vi "fuzz.vi"() -> ()   [LabVIEW 2025]
panel:
  in  "Boolean 4":bool
  out "output array 6":dbl[][](array[numeric])
  out "output array 5":dbl[][](array[numeric])
  out "output array 4":dbl[][](array[numeric])
  out "output array 3":dbl[][](array[numeric])
  out "output array 2":dbl[][](array[numeric])
  out "output array":dbl[][](array[numeric])
  out "1-D Array of Real":dbl[](array[numeric])
  in  "stop 2":bool
  in  "Boolean 3":bool
  in  "Boolean 2":bool
  in  "Boolean":bool
  out "String 6":string
  out "String 5":string
  out "String 4":string
  out "String 3":string
  out "String 2":string
  out "IM6":picture
  out "IM5":picture
  out "IM4":picture
  out "IM3":picture
  out "IM2":picture
  out "Numeric":i32
  out "Real":dbl
  out "String":string
  out "?":picture
  in  "Evaluate":path
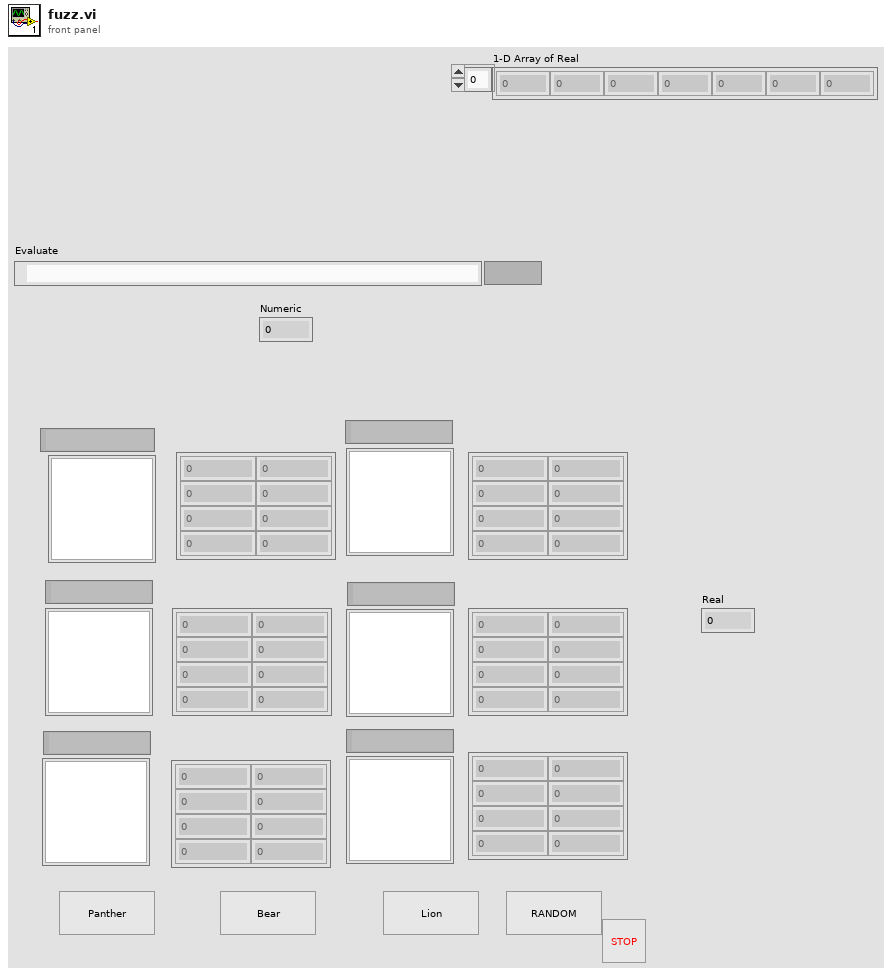
[diagram p1: front panel]
types:
  T1 = typedef "imagedata.ctl" = cluster{"image type":i32, "image depth":i32, "image":u8[], "mask":u8[], "colors":u32[], "Rectangle":cluster{"left":i16, "top":i16, "right":i16, "bottom":i16}}
  T2 = typedef "LVBoundsTypeDef.ctl" = cluster{"Width":u32, "Height":u32}
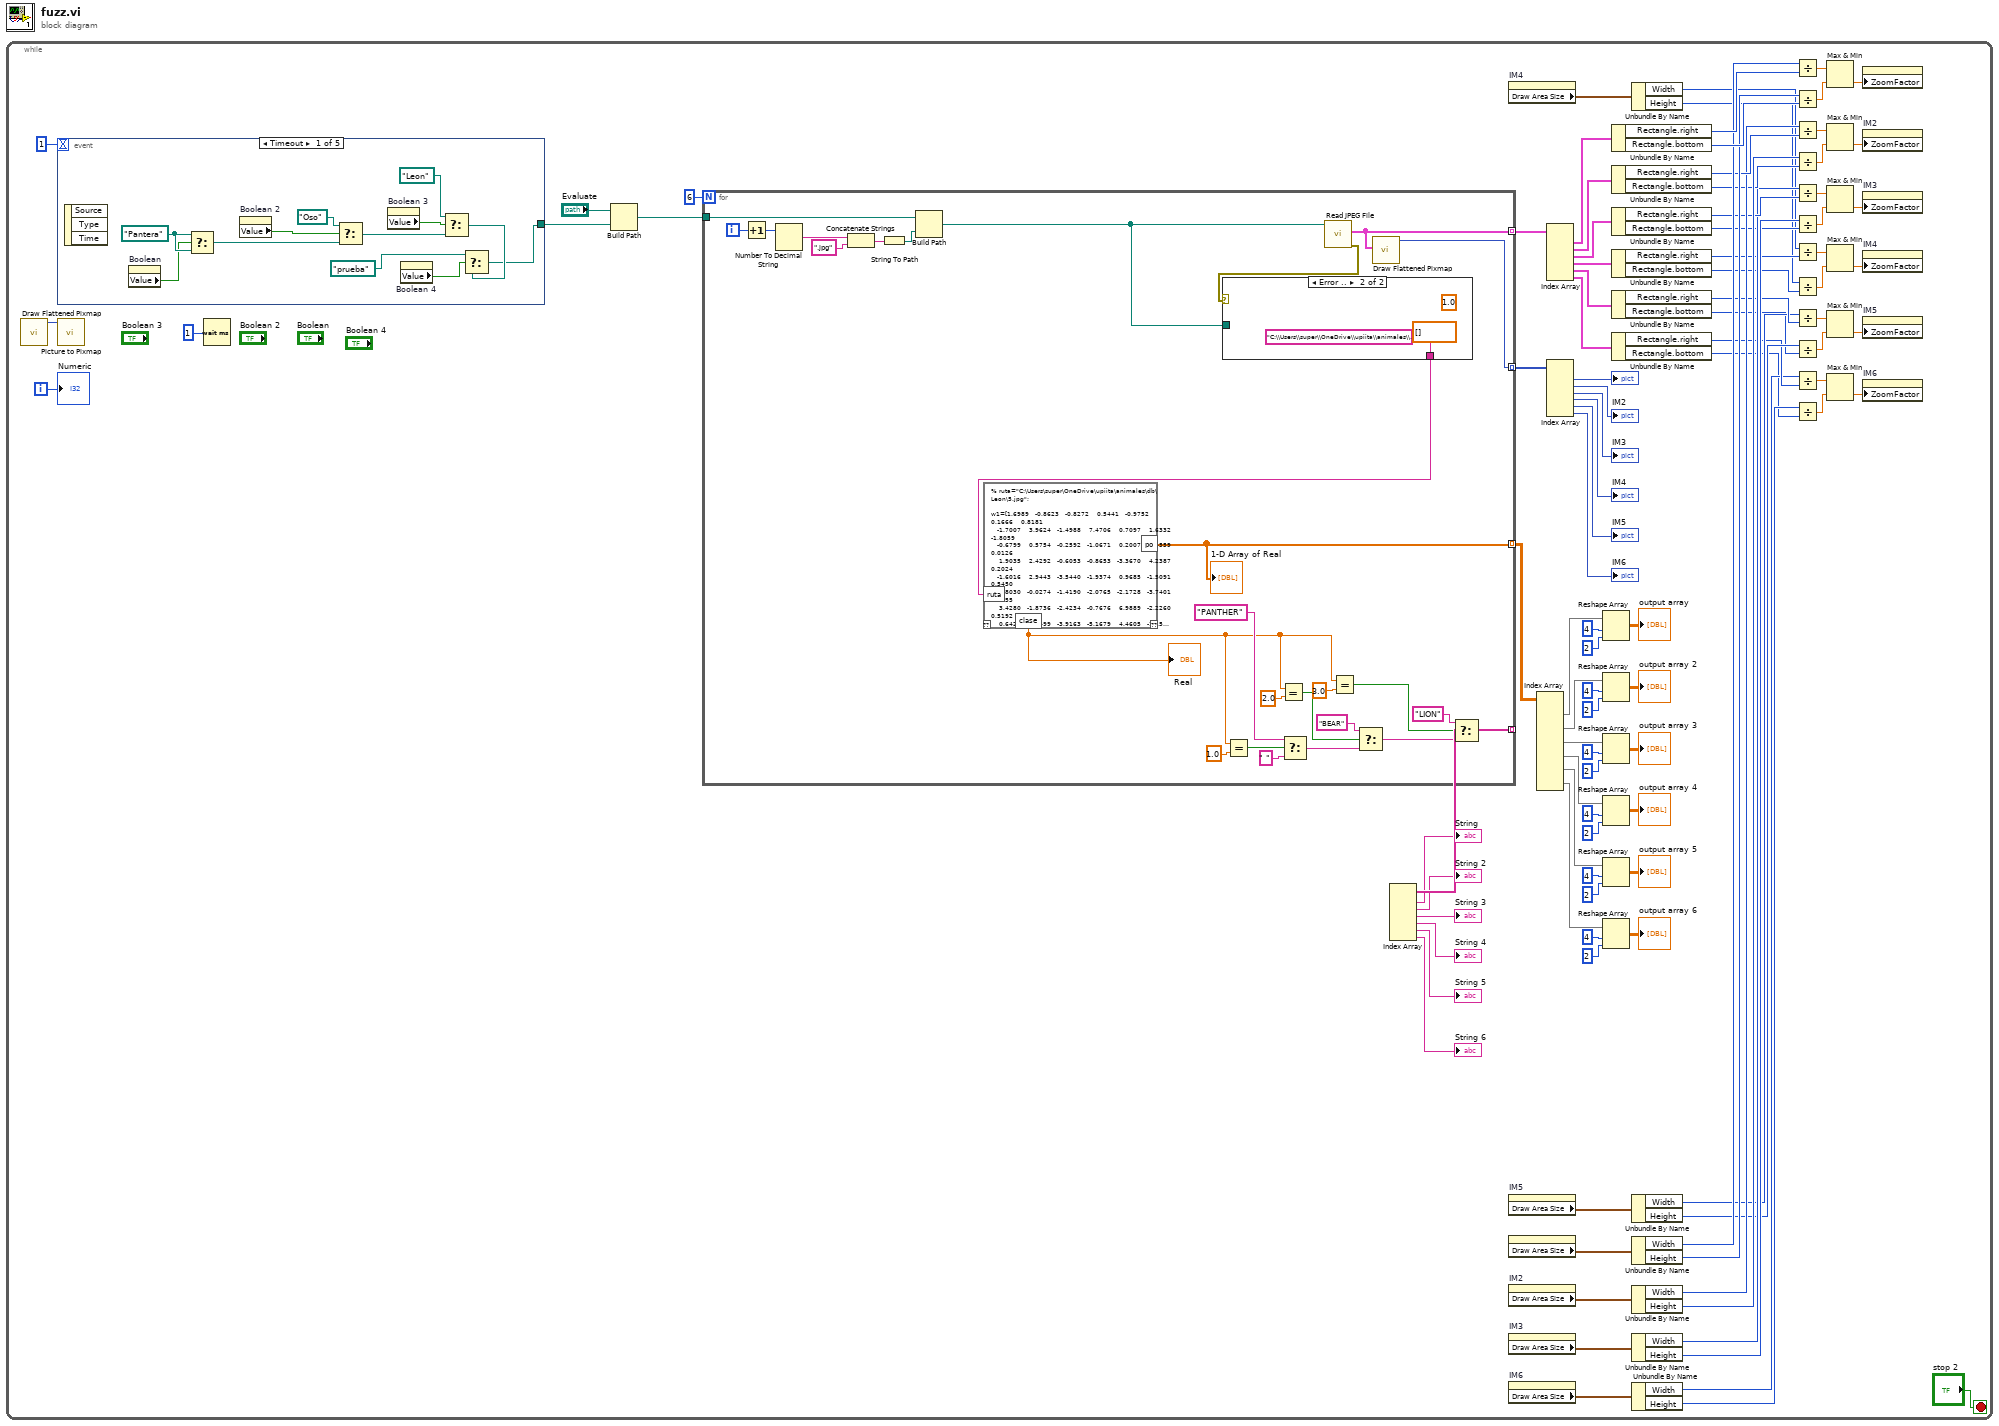
[diagram p0: block diagram]
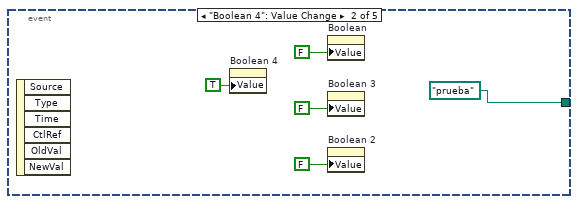
[diagram p2: hidden frame]
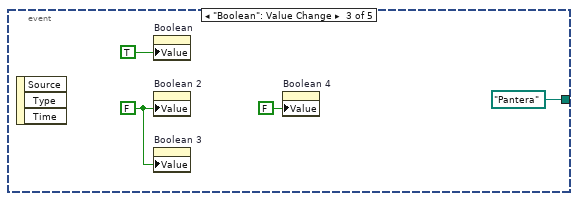
[diagram p3: hidden frame]
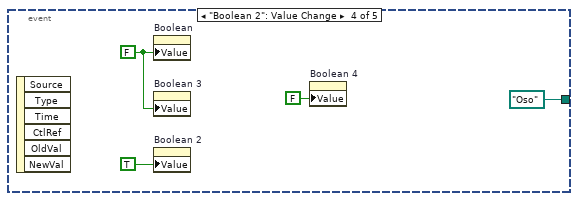
[diagram p4: hidden frame]
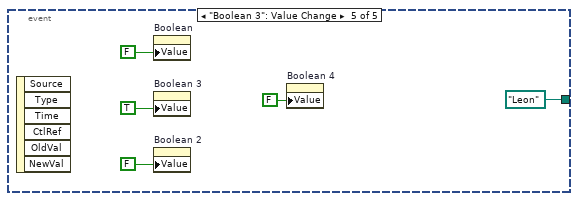
[diagram p5: hidden frame]
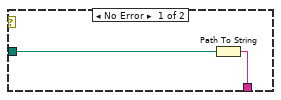
[diagram p6: hidden frame]
diagram:
  n1 = while {
    i -> [w103]
    stop <- "stop 2" stop-if-true
    n2 = call <vilib>:"Draw Flattened Pixmap.vi"() -> ("new picture"=w95:picture)  [unwired: 9 in]
    n3 = event shown="[0] Timeout" {
      selector: _ -> [_ _ _ _ _]
      dyn-events: _ -> [_ _ _ _ _]
      timeout: 1 -> [_ _ _ _ _]
      tunnel: [w104 path "prueba" ("Evaluate") path "Pantera" ("Evaluate") path "Oso" ("Evaluate") path "Leon" ("Evaluate")] -> w28
      event Timeout {
        w109 = path "Pantera" ("Evaluate")
        n4 = event-data() -> ()  [unwired: 1 in, 3 out]
        n5 = property on="Boolean" class="Bool (strict)"() -> ("Value"=w108:bool)  [unwired: 2 in, 2 out]
        n6 = Select(t=w109, s=w108, f=w109) -> (s? t:f=w113:path)
        n7 = property on="Boolean 2" class="Bool (strict)"() -> ("Value"=w112:bool)  [unwired: 2 in, 2 out]
        n8 = Select(t=path "Oso" ("Evaluate"), s=w112, f=w113) -> (s? t:f=w115:path)
        n9 = property on="Boolean 3" class="Bool (strict)"() -> ("Value"=w114:bool)  [unwired: 2 in, 2 out]
        n10 = property on="Boolean 4" class="Bool (strict)"() -> ("Value"=w107:bool)  [unwired: 2 in, 2 out]
        n11 = Select(t=path "Leon" ("Evaluate"), s=w114, f=w115) -> (s? t:f=w105:path)
        n12 = Select(t=path "prueba" ("Evaluate"), s=w107, f=w105) -> (s? t:f=w104:path)
      }
      event "Boolean 4": Value Change {
        n13 = event-data() -> ()  [unwired: 1 in, 6 out]
        n14 = property on="Boolean 4" class="Bool (strict)"("Value"=TRUE ("Boolean 4")) -> ()  [unwired: 2 in, 2 out]
        n15 = property on="Boolean" class="Bool (strict)"("Value"=FALSE) -> ()  [unwired: 2 in, 2 out]
        n16 = property on="Boolean 3" class="Bool (strict)"("Value"=FALSE) -> ()  [unwired: 2 in, 2 out]
        n17 = property on="Boolean 2" class="Bool (strict)"("Value"=FALSE) -> ()  [unwired: 2 in, 2 out]
      }
      event "Boolean": Value Change {
        w124 = FALSE
        n18 = event-data() -> ()  [unwired: 1 in, 3 out]
        n19 = property on="Boolean" class="Bool (strict)"("Value"=TRUE) -> ()  [unwired: 2 in, 2 out]
        n20 = property on="Boolean 2" class="Bool (strict)"("Value"=w124) -> ()  [unwired: 2 in, 2 out]
        n21 = property on="Boolean 3" class="Bool (strict)"("Value"=w124) -> ()  [unwired: 2 in, 2 out]
        n22 = property on="Boolean 4" class="Bool (strict)"("Value"=FALSE ("Boolean 4")) -> ()  [unwired: 2 in, 2 out]
      }
      event "Boolean 2": Value Change {
        w128 = FALSE
        n23 = event-data() -> ()  [unwired: 1 in, 6 out]
        n24 = property on="Boolean" class="Bool (strict)"("Value"=w128) -> ()  [unwired: 2 in, 2 out]
        n25 = property on="Boolean 3" class="Bool (strict)"("Value"=w128) -> ()  [unwired: 2 in, 2 out]
        n26 = property on="Boolean 2" class="Bool (strict)"("Value"=TRUE) -> ()  [unwired: 2 in, 2 out]
        n27 = property on="Boolean 4" class="Bool (strict)"("Value"=FALSE ("Boolean 4")) -> ()  [unwired: 2 in, 2 out]
      }
      event "Boolean 3": Value Change {
        n28 = event-data() -> ()  [unwired: 1 in, 6 out]
        n29 = property on="Boolean" class="Bool (strict)"("Value"=FALSE) -> ()  [unwired: 2 in, 2 out]
        n30 = property on="Boolean 3" class="Bool (strict)"("Value"=TRUE) -> ()  [unwired: 2 in, 2 out]
        n31 = property on="Boolean 2" class="Bool (strict)"("Value"=FALSE) -> ()  [unwired: 2 in, 2 out]
        n32 = property on="Boolean 4" class="Bool (strict)"("Value"=FALSE ("Boolean 4")) -> ()  [unwired: 2 in, 2 out]
      }
    }
    n33 = call <vilib>:"Picture to Pixmap.vi"("picture"=w95) -> ()  [unwired: 9 in, 2 out]
    n34 = Wait (ms)(milliseconds to wait=u32 1) -> ()  [unwired: 1 out]
    n35 = Build Path(base path="Evaluate", name or relative path=w28) -> (appended path=w29:path)
    n36 = for {
      N: 6 -> [_]
      tunnel: [w141] -> w102 mode=indexing
      tunnel: [w140] -> w86 mode=indexing
      tunnel: [w139] -> w84 mode=indexing
      tunnel: w29 -> [w138]
      tunnel: [w136] -> w26 mode=indexing
      i -> [w147]
      n37 = Increment(x=w147) -> (x+1=w146:i32)
      n38 = Number To Decimal String(number=w146) -> (decimal integer string=w145:string)  [unwired: 1 in]
      n39 = Concatenate Strings(w145, ".jpg" ("string")) -> (w142:string)
      n40 = String To Path(string=w142) -> (path=w143:path)
      n41 = Build Path(base path=w138, name or relative path=w143) -> (appended path=w135:path)
      n42 = call <vilib>:"Read JPEG File.vi"("path to JPEG file"=w135) -> ("error out"=w160:errorcluster, "image data"=w140:T1)  [unwired: 8 in, 1 out]
      n43 = case shown="Error .." w160 {
        tunnel: w135 -> [w162 _]
        tunnel: [w161 "C:\\Users\\super\\OneDrive\\upiita\\animales\\Pantera\\2.jpg"] -> w134
        frame No Error {
          n44 = Path To String(path=w162) -> (string=w161:string)
        }
        frame Error {
          (unwired) 1.0
          (unwired) dbl[] []
        }
      }
      n45 = script code="% ruta=\"C:\\Users\\super\\OneDrive\\upiita\\animales\\db\\Leon\\5.jpg\";\n\nw1=[1.6989   -0.8623   -0.8272    0.5441   -0.9752    0.1666    0.8181\n   -1.7007    3.9624   -1.4988    7.4706    0.7097    1.6332   -1.8059\n   -0.6799    0.5754   -0.2592   -1.0671    0.2007    0.4559    0.0126\n    1.9035    2.4292   -0.6053   -0.8653   -3.3670    4.2387    0.2024\n   -1.6016    2.9443   -3.5440   -1.9374    0.9685   -1.5091    0.5450\n    1.8030   -0.0274   -1.4190   -2.0765   -2.1728   -3.7401    3.2655\n    3.4280   -1.8736   -2.4234   -0.7676    6.9889   -2.2260    0.5192\n    0.6423    3.7499   -3.9163   -5.1679    4.4605   -1.1594    1.2309\n    0.7221   -2.7849    1.5068   -0.3904    3.3638   -3.1946   -1.1201\n    0.1992    4.7957    1.9419    4.5777   -5.3795    0.3820    1.6822\n    0.1973    1.9907    0.5992    0.9223   -0.2957    0.0360   -0.0986\n   -2.8224    8.8552    1.9215   -4.5294   -0.7394    0.3050   -7.3801\n   -1.8354   -0.4141    1.8706   -3.3358    2.7823    1.3767   -2.8708\n   -2.4730    1.6603    0.1048   -1.4714    0.1605   -1.1670    0.9838\n    1.3272   -0.6674    0.3132    4.4050   -3.8333   -1.0422    0.7726\n    0.1146   -3.9097    2.8094   -4.6702   -1.4831   -0.3201    1.0435\n    0.6448  -12.2911   -9.3138    1.8255    0.4273    4.6842   -0.0133\n   -0.3258    2.3390   -1.6407   -0.3822   -2.9938    3.6387    0.9024\n    0.0543    1.6570    0.5888    0.8988   -0.7652   -0.6278    0.6053\n    1.4302   10.2594    6.4344   -0.3511   -1.0367   -0.1546   -1.4964\n    0.9887    0.0115   -1.1112    1.0604   -1.1970   -0.5493    1.6300\n   -0.2303    0.7127    0.8553   -1.6591   -2.4578    1.0508   -2.0880\n    0.2508    2.1277   -1.0004   -3.0484    2.9977   -0.4361    1.1811\n    0.0827    3.7358    0.8479    1.2354   -0.8090   -1.4833    0.3593\n   -4.1841   -2.2305    0.8204   -1.1749   -3.6980    0.6915    0.9924\n    ];\nw21=[1.9587   -0.3172    2.0654\n    1.6334   -7.3767    6.6522\n   -1.1411    0.1939   -1.2969\n   -4.0234    5.3367   -2.8570\n   -6.4760    0.5986   -0.5273\n   -1.6462   -4.6876    5.9580\n    3.2146    6.4110   -4.9817\n   -7.8278    5.2316   -6.8578\n    2.3145   -5.1749    2.6464\n   -8.9091    3.0109    2.3905\n   -1.5185   -1.8959   -0.0938\n   -8.2801    0.9810    6.8302\n   -2.5548    3.0711   -7.5759\n   -4.2162   -0.1662   -0.6635\n    3.6889   -6.1318    1.2892\n    3.4382    4.8346   -4.3151\n   10.1588    1.5537   -9.1353\n   -2.5363    4.4542   -2.9463\n   -1.3802   -1.5687    0.9607\n   -6.0826   -3.0323    7.8469\n    1.1507   -1.1190    3.0469\n    3.6294   -0.4964   -4.9489\n   -0.1919    1.5799   -5.2593\n   -2.8139   -2.6355    1.6323\n    5.3808   -2.4561    1.5991\n  ];\nw2=w21';\nb1=[-0.7617\n   -2.8060\n    0.1299\n   -0.6007\n    0.1556\n    2.0319\n   -3.4328\n   -0.5864\n   -0.0923\n    1.6977\n   -0.4547\n    0.5667\n    1.6589\n    0.8048\n    2.2292\n    0.4752\n    0.3909\n   -0.1661\n    0.2171\n    3.1523\n   -1.0838\n   -2.6712\n   -0.7240\n    0.8969\n   -1.3636];\nb2=[-0.2438\n   -0.1909\n    0.1054\n\n    ];\nmu=[0.2001\n    0.0581\n    2.9434\n    0.6793\n    0.0940\n   15.4709\n    0.5379];\nsigma=[0.3182\n    0.0741\n    0.0710\n    0.1435\n    0.0732\n    8.3950\n    0.2413\n    ];\n\nI = imread(ruta);\nIgray = rgb2gray(I);\nIbin = imbinarize(Igray);\n\nIhsv = rgb2hsv(I);\npixelsHSV = reshape(Ihsv(repmat(Ibin,[1 1 3])),[],3);\n\nHmean = mean(pixelsHSV(:,1));\nSmean = mean(pixelsHSV(:,2));\nVmean = mean(pixelsHSV(:,3));\n\narea = sum(Ibin(:));\nareaNorm = area / numel(Ibin);\n\nper = sum(bwperim(Ibin),'all');\nperNorm = per / sqrt(area);\n\ncircularidad = 4*pi*area/(per^2);\n\nstats = regionprops(Ibin,'Area','Eccentricity');\n[~,idx] = max([stats.Area]);\necc = stats(idx).Eccentricity;\n\nPt_test = [Hmean; Smean; Vmean; areaNorm; circularidad; perNorm; ecc];\nPt_test = (Pt_test - mu) ./ sigma;\n\na1 = logsig(w1*Pt_test + b1);\na2 = logsig(w2*a1 + b2);\n\n[~,clase] = max(a2);\nclase"("ruta"=w134) -> ("clase"=w137:dbl, "po"=w136:dbl[])  [unwired: 1 in, 1 out]
      "Real" <- w137
      "1-D Array of Real" <- w136
      n46 = Equal?(x=w137, y=1.0) -> (x = y?=w158:bool)
      n47 = Equal?(x=w137, y=2.0) -> (x = y?=w155:bool)
      n48 = Select(t="PANTHER", s=w158, f=" ") -> (s? t:f=w153:string)
      n49 = Equal?(x=w137, y=3.0) -> (x = y?=w150:bool)
      n50 = Select(t="BEAR", s=w155, f=w153) -> (s? t:f=w149:string)
      n51 = call <vilib>:"Draw Flattened Pixmap.vi"("image data"=w140) -> ("new picture"=w139:picture)  [unwired: 8 in]
      n52 = Select(t="LION", s=w150, f=w149) -> (s? t:f=w141:string)
    }
    n53 = Index Array(array=w102) -> (element #1=→"String":string, element #2=→"String 2":string, element #3=→"String 3":string, element #4=→"String 4":string, element #5=→"String 5":string, element #6=→"String 6":string)  [unwired: 6 in]
    n54 = property on="IM4" class="Pict"() -> ("Draw Area Size"=w53:T2)  [unwired: 2 in, 2 out]
    n55 = property on="IM5" class="Pict"() -> ("Draw Area Size"=w44:T2)  [unwired: 2 in, 2 out]
    n56 = property class="Pict"() -> ("Draw Area Size"=w87:T2)  [unwired: 2 in, 2 out]
    n57 = property on="IM2" class="Pict"() -> ("Draw Area Size"=w77:T2)  [unwired: 2 in, 2 out]
    n58 = property on="IM3" class="Pict"() -> ("Draw Area Size"=w62:T2)  [unwired: 2 in, 2 out]
    n59 = property on="IM6" class="Pict"() -> ("Draw Area Size"=w35:T2)  [unwired: 2 in, 2 out]
    n60 = Index Array(array=w26) -> (element #1=w25:dbl[], element #2=w5:dbl[], element #3=w4:dbl[], element #4=w3:dbl[], element #5=w2:dbl[], element #6=w1:dbl[])  [unwired: 12 in]
    n61 = Index Array(array=w86) -> (element #1=w85:T1, element #2=w76:T1, element #3=w60:T1, element #4=w51:T1, element #5=w42:T1, element #6=w33:T1)  [unwired: 6 in]
    n62 = Index Array(array=w84) -> (element #1=→"?":picture, element #2=→"IM2":picture, element #3=→"IM3":picture, element #4=→"IM4":picture, element #5=→"IM5":picture, element #6=→"IM6":picture)  [unwired: 6 in]
    n63 = Reshape Array(w25, 4 ("dimension size"), 2 ("dimension size")) -> (→"output array":dbl[][])
    n64 = Reshape Array(w5, 4 ("dimension size"), 2 ("dimension size")) -> (→"output array 2":dbl[][])
    n65 = Reshape Array(w4, 4 ("dimension size"), 2 ("dimension size")) -> (→"output array 3":dbl[][])
    n66 = Reshape Array(w3, 4 ("dimension size"), 2 ("dimension size")) -> (→"output array 4":dbl[][])
    n67 = Reshape Array(w2, 4 ("dimension size"), 2 ("dimension size")) -> (→"output array 5":dbl[][])
    n68 = Reshape Array(w1, 4 ("dimension size"), 2 ("dimension size")) -> (→"output array 6":dbl[][])
    n69 = Unbundle By Name(w85) -> ("Rectangle.right"=w94:i16, "Rectangle.bottom"=w93:i16)
    n70 = Unbundle By Name(w76) -> ("Rectangle.right"=w83:i16, "Rectangle.bottom"=w75:i16)
    n71 = Unbundle By Name(w60) -> ("Rectangle.right"=w68:i16, "Rectangle.bottom"=w61:i16)
    n72 = Unbundle By Name(w51) -> ("Rectangle.right"=w59:i16, "Rectangle.bottom"=w52:i16)
    n73 = Unbundle By Name(w42) -> ("Rectangle.right"=w50:i16, "Rectangle.bottom"=w43:i16)
    n74 = Unbundle By Name(w33) -> ("Rectangle.right"=w41:i16, "Rectangle.bottom"=w34:i16)
    n75 = Unbundle By Name(w53) -> ("Width"=w57:u32, "Height"=w58:u32)
    n76 = Unbundle By Name(w44) -> ("Width"=w48:u32, "Height"=w49:u32)
    n77 = Unbundle By Name(w87) -> ("Width"=w91:u32, "Height"=w92:u32)
    n78 = Unbundle By Name(w77) -> ("Width"=w81:u32, "Height"=w82:u32)
    n79 = Unbundle By Name(w62) -> ("Width"=w66:u32, "Height"=w67:u32)
    n80 = Unbundle By Name(w35) -> ("Width"=w39:u32, "Height"=w40:u32)
    n81 = Divide(x=w91, y=w94) -> (x/y=w88:dbl)
    n82 = Divide(x=w92, y=w93) -> (x/y=w89:dbl)
    n83 = Divide(x=w81, y=w83) -> (x/y=w78:dbl)
    n84 = Divide(x=w82, y=w75) -> (x/y=w79:dbl)
    n85 = Divide(x=w66, y=w68) -> (x/y=w63:dbl)
    n86 = Divide(x=w67, y=w61) -> (x/y=w64:dbl)
    n87 = Divide(x=w57, y=w59) -> (x/y=w54:dbl)
    n88 = Divide(x=w58, y=w52) -> (x/y=w55:dbl)
    n89 = Divide(x=w48, y=w50) -> (x/y=w45:dbl)
    n90 = Divide(x=w49, y=w43) -> (x/y=w46:dbl)
    n91 = Divide(x=w39, y=w41) -> (x/y=w36:dbl)
    n92 = Divide(x=w40, y=w34) -> (x/y=w37:dbl)
    n93 = Max & Min(x=w88, y=w89) -> (min(x,y)=w90:dbl)  [unwired: 1 out]
    n94 = Max & Min(x=w78, y=w79) -> (min(x,y)=w80:dbl)  [unwired: 1 out]
    n95 = Max & Min(x=w63, y=w64) -> (min(x,y)=w65:dbl)  [unwired: 1 out]
    n96 = Max & Min(x=w54, y=w55) -> (min(x,y)=w56:dbl)  [unwired: 1 out]
    n97 = Max & Min(x=w45, y=w46) -> (min(x,y)=w47:dbl)  [unwired: 1 out]
    n98 = Max & Min(x=w36, y=w37) -> (min(x,y)=w38:dbl)  [unwired: 1 out]
    n99 = property class="Pict"("ZoomFactor"=w90) -> ()  [unwired: 2 in, 2 out]
    n100 = property on="IM2" class="Pict"("ZoomFactor"=w80) -> ()  [unwired: 2 in, 2 out]
    n101 = property on="IM3" class="Pict"("ZoomFactor"=w65) -> ()  [unwired: 2 in, 2 out]
    n102 = property on="IM4" class="Pict"("ZoomFactor"=w56) -> ()  [unwired: 2 in, 2 out]
    n103 = property on="IM5" class="Pict"("ZoomFactor"=w47) -> ()  [unwired: 2 in, 2 out]
    n104 = property on="IM6" class="Pict"("ZoomFactor"=w38) -> ()  [unwired: 2 in, 2 out]
    "Numeric" <- w103
  }
